vi "DAQ Assist Output.vi"(7 "index":i32) -> ()   [LabVIEW 2015]
panel:
  in  "data":u32[](array[numeric])=[128, 144, 192, 160, 161, 162, 163, 164, 0, 0, 0, 0]
  in  "device name":tag="Dev2"
  out "error out":errorcluster
  in  "error in":errorcluster
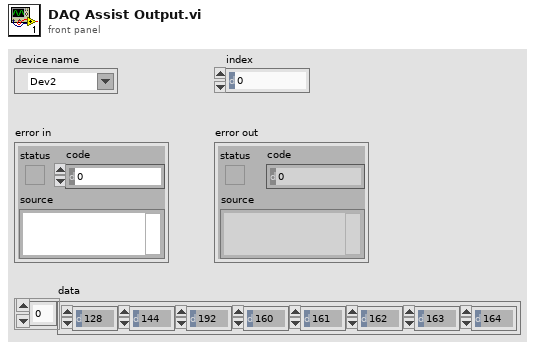
[diagram p1: front panel]
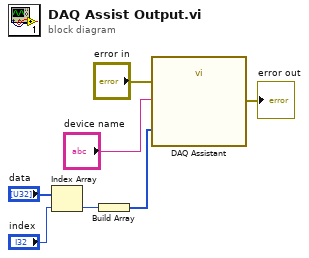
[diagram p0: block diagram]
diagram:
  n1 = Index Array(array="data", index="index") -> (element=w4:u32)
  n2 = Build Array(w4) -> (w1:u32[])
  n3 = call "DAQ Assistant"("data"=w1, "error in"="error in", "device name"="device name") -> ("error out"=→"error out":errorcluster)  [unwired: 15 in, 1 out]
